vi "Day9-1.vi"() -> ()   [LabVIEW 2021]
panel:
  out "Tail pos":cluster{"x":i32, "y":i32}[](array[cluster])
  out "Head pos":cluster{"x":i32, "y":i32}[](array[cluster])
  out "size":i32
  out "Array":string[](array[string])
  out "array":string[][](array[string])
  in  "Tail":cluster{"x":i32, "y":i32}
  in  "Head":cluster{"x":i32, "y":i32}
  out "tail position":cluster{"x":i32, "y":i32}
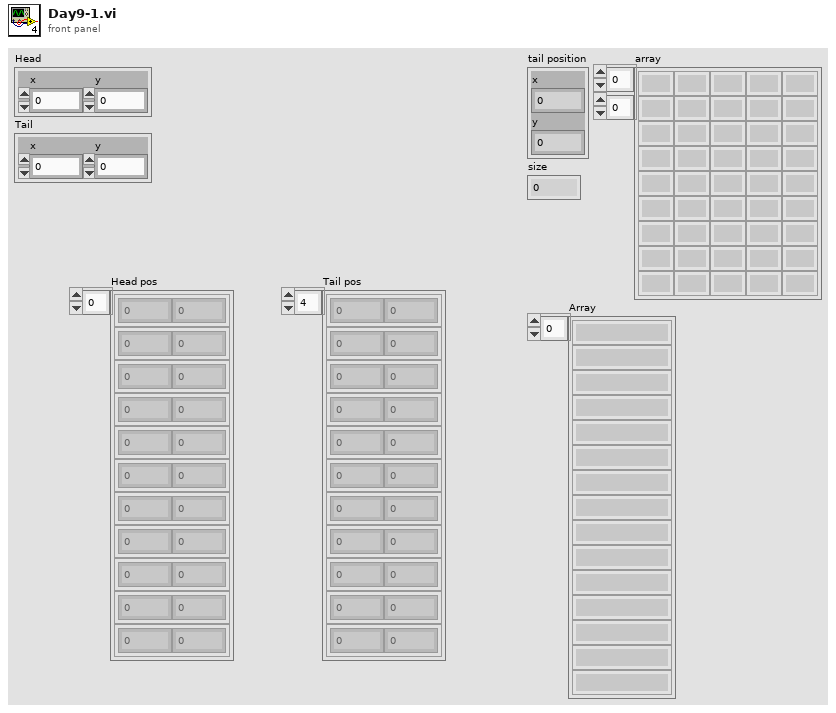
[diagram p1: front panel]
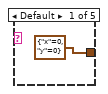
[diagram p2: hidden frame]
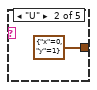
[diagram p3: hidden frame]
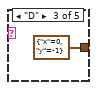
[diagram p4: hidden frame]
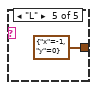
[diagram p5: hidden frame]
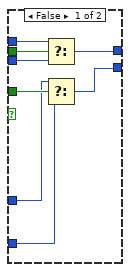
[diagram p6: hidden frame]
diagram:
  w8 = set{cluster{"x":i32, "y":i32}} {}  # Size: 0
  # "Initial starting position of Head and Tail = (0,0)"
  n1 = Spreadsheet String To Array(delimiter (Tab)=" ", format string="%s", spreadsheet string="R 2\nD 2\nR 2\nU 1\nR 2\nL 2\nD 1\nL 1\nD 2\nR 2\nU 2\nD 1\nR 2\nD 2\nU 1\nR 1\nD 1\nL 1\nU 1\nR 1\nL 1\nR 2\nU 2\nD 2\nR 2\nL 2\nU 1\nL 2\nU 2\nL 2\nR 2\nU 2\nR 1\nU 2\nL 2\nD 1\nR 1\nU 2\nD 2\nR 2\nL 2\nU 1\nD 1\nL 2\nU 2\nL 2\nU 1\nD 2\nR 1\nD 1\nR 2\nU 1\nL 2\nD 1\nU 2\nR 2\nL 1\nD 2\nU 1\nD 1\nL 1\nU 1\nR 1\nD 1\nR 1\nU 1\nD 2\nL 1\nD 1\nR 2\nD 1\nU 2\nD 2\nU 2\nL 1\nU 2\nR 2\nL 2\nD 2\nR 1\nL 2\nU 2\nL 1\nU 1\nL 1\nR 2\nL 2\nR 1\nD 1\nU 1\nL 2\nR 1\nL 1\nU 1\nD 1\nU 1\nD 1\nR 1\nL 2\nR 2\nL 1\nU 1\nD 2\nU 2\nL 2\nR 2\nU 1\nR 2\nL 2\nR 2\nL 1\nU 3\nD 1\nL 1\nD 3\nU 1\nD 2\nL 1\nR 3\nD 2\nU 3\nR 1\nD 3\nR 2\nD 1\nU 3\nL 1\nR 2\nL 3\nD 3\nU 2\nL 2\nR 3\nU 3\nD 3\nL 3\nD 2\nL 3\nR 1\nL 1\nD 1\nU 3\nD 3\nU 2\nL 3\nR 3\nU 1\nD 2\nR 2\nL 2\nD 3\nR 3\nU 1\nR 1\nL 3\nU 2\nL 2\nU 1\nR 1\nD 1\nR 3\nU 2\nD 1\nL 1\nU 1\nR 2\nL 1\nR 3\nL 1\nU 3\nL 2\nD 2\nL 2\nD 3\nL 2\nR 1\nU 2\nL 3\nD 1\nL 3\nD 1\nU 2\nL 3\nR 2\nU 1\nL 3\nD 3\nR 3\nU 2\nR 2\nD 3\nR 3\nU 2\nR 2\nL 2\nU 3\nR 1\nL 2\nD 3\nU 1\nL 1\nU 1\nL 2\nR 3\nL 3\nD 3\nR 3\nU 3\nL 1\nR 2\nD 3\nU 1\nR 2\nU 1\nD 1\nL 1\nD 2\nL 2\nD 3\nU 2\nD 1\nU 3\nD 3\nU 3\nR 3\nL 3\nU 4\nL 3\nD 1\nR 4\nU 3\nD 2\nR 1\nD 4\nL 3\nU 1\nL 1\nR 2\nD 1\nR 3\nD 3\nL 3\nD 4\nL 3\nR 4\nU 3\nR 3\nD 1\nR 3\nD 3\nR 3\nD 4\nU 4\nR 2\nD 3\nR 3\nD 2\nU 1\nR 2\nD 2\nU 2\nD 3\nL 2\nR 4\nD 4\nU 4\nR 3\nU 4\nR 1\nU 2\nR 4\nD 2\nL 4\nR 4\nU 3\nL 2\nU 2\nL 3\nR 3\nL 1\nU 4\nL 3\nU 3\nL 3\nU 1\nR 2\nU 3\nR 2\nL 3\nU 1\nD 3\nR 4\nD 1\nR 2\nL 1\nD 1\nU 2\nD 3\nR 4\nU 1\nL 3\nR 4\nU 4\nL 4\nR 2\nD 1\nU 4\nR 1\nD 3\nL 3\nD 1\nR 3\nD 2\nU 2\nL 1\nU 2\nD 3\nL 1\nU 3\nD 3\nL 3\nU 2\nL 3\nU 2\nR 1\nD 1\nR 1\nL 1\nD 2\nR 3\nD 2\nL 2\nR 3\nD 5\nR 5\nU 4\nD 5\nU 5\nD 4\nR 4\nD 2\nR 5\nL 4\nR 2\nL 2\nR 5\nU 5\nR 1\nD 2\nR 1\nL 3\nD 5\nU 3\nD 4\nR 3\nU 4\nD 1\nU 4\nL 5\nR 1\nU 4\nL 5\nU 3\nD 4\nL 2\nD 4\nU 4\nL 2\nD 1\nR 3\nD 1\nR 2\nD 4\nR 5\nL 1\nU 4\nL 4\nU 3\nL 1\nU 1\nR 4\nU 3\nL 1\nR 3\nD 5\nU 2\nR 4\nD 3\nL 2\nD 4\nR 5\nD 2\nU 3\nR 4\nD 4\nL 2\nU 4\nR 5\nL 1\nU 5\nD 1\nR 3\nL 4\nD 1\nU 3\nD 5\nR 2\nD 2\nL 5\nU 2\nD 3\nL 5\nD 5\nL 1\nR 5\nD 2\nU 3\nR 2\nL 2\nU 1\nL 5\nR 1\nL 4\nD 5\nR 5\nD 2\nU 5\nL 5\nD 1\nL 1\nD 3\nR 1\nD 2\nL 2\nR 4\nU 5\nL 2\nR 1\nU 3\nD 1\nU 1\nD 5\nR 2\nD 2\nR 3\nD 6\nU 1\nR 6\nD 4\nU 1\nR 5\nL 6\nR 2\nL 6\nU 6\nR 5\nD 2\nU 1\nD 2\nL 2\nD 5\nR 3\nU 4\nD 2\nL 1\nU 1\nD 3\nU 1\nD 1\nR 5\nU 1\nR 1\nD 3\nU 5\nL 6\nR 3\nL 6\nU 4\nD 2\nR 1\nL 6\nR 2\nD 3\nU 2\nR 2\nL 1\nD 1\nU 1\nR 4\nU 1\nR 2\nU 2\nL 2\nU 2\nD 5\nL 4\nU 6\nL 3\nD 6\nU 5\nL 6\nU 3\nR 5\nU 2\nR 4\nL 6\nD 1\nR 5\nD 4\nL 2\nR 2\nU 1\nD 2\nL 2\nU 4\nR 1\nD 2\nU 2\nR 6\nL 2\nD 5\nR 5\nL 3\nD 1\nU 1\nL 2\nD 4\nR 6\nL 5\nR 3\nU 1\nR 3\nL 1\nR 3\nU 1\nL 1\nU 4\nD 4\nU 3\nR 3\nU 1\nR 2\nD 1\nL 6\nU 2\nR 2\nD 1\nR 5\nL 2\nD 5\nL 3\nR 6\nD 2\nL 2\nD 3\nL 5\nD 7\nL 7\nD 4\nU 5\nR 7\nL 7\nD 3\nU 5\nR 6\nU 3\nL 6\nR 5\nL 4\nD 4\nR 4\nL 6\nD 6\nU 3\nD 3\nR 7\nU 1\nL 5\nU 3\nL 4\nU 3\nL 5\nD 1\nR 7\nU 3\nL 6\nD 1\nU 3\nL 2\nU 6\nL 6\nD 1\nU 1\nD 2\nL 5\nU 4\nR 5\nD 7\nU 3\nD 4\nL 1\nD 3\nR 7\nD 2\nU 4\nL 1\nD 3\nR 3\nD 6\nR 4\nU 3\nD 4\nR 6\nL 7\nU 5\nL 7\nR 3\nL 7\nD 5\nR 7\nD 4\nU 3\nR 6\nU 7\nD 2\nR 2\nL 2\nD 1\nR 3\nU 3\nD 5\nU 3\nL 3\nD 6\nL 6\nR 1\nL 5\nD 6\nU 4\nR 2\nL 2\nD 1\nU 7\nL 5\nD 3\nU 1\nL 1\nR 1\nL 6\nR 1\nD 6\nU 4\nL 7\nU 6\nR 6\nL 2\nD 5\nR 1\nD 6\nL 1\nR 3\nD 1\nU 5\nL 1\nD 3\nU 7\nD 5\nU 7\nD 7\nU 4\nR 3\nU 4\nL 8\nU 1\nR 1\nD 2\nU 5\nD 2\nL 5\nD 6\nU 4\nR 5\nL 5\nU 7\nL 3\nD 1\nL 2\nR 8\nL 1\nU 8\nL 2\nD 3\nR 6\nL 8\nD 2\nL 1\nU 4\nD 1\nR 2\nD 7\nU 5\nD 4\nU 4\nL 2\nD 6\nU 1\nD 5\nU 2\nD 2\nL 8\nD 6\nL 2\nU 1\nR 7\nD 1\nU 5\nL 6\nD 3\nL 2\nD 8\nR 6\nL 5\nU 2\nL 6\nU 4\nD 6\nL 7\nU 8\nL 5\nD 8\nR 8\nD 6\nL 3\nU 6\nL 1\nD 8\nR 7\nL 7\nR 2\nD 6\nR 1\nU 5\nL 5\nR 5\nL 3\nU 8\nL 1\nU 2\nD 5\nR 8\nU 5\nL 5\nD 2\nR 5\nU 1\nD 8\nR 3\nU 1\nR 6\nD 6\nR 5\nD 6\nL 8\nU 8\nL 8\nU 8\nL 8\nR 8\nU 8\nR 5\nL 1\nD 3\nU 1\nD 6\nU 1\nL 8\nU 3\nR 5\nL 2\nR 1\nD 2\nL 2\nU 4\nD 1\nR 1\nD 2\nR 2\nU 4\nR 3\nU 8\nD 9\nL 9\nD 5\nL 4\nD 7\nL 9\nU 4\nL 9\nD 7\nU 4\nL 3\nU 2\nR 5\nU 3\nL 1\nR 5\nL 8\nU 4\nR 6\nL 8\nU 1\nR 7\nD 6\nR 6\nU 7\nL 9\nR 7\nU 8\nR 5\nU 6\nL 4\nD 4\nL 3\nR 8\nU 6\nL 7\nR 4\nD 7\nR 3\nL 3\nD 2\nL 2\nU 5\nR 8\nL 7\nR 9\nD 8\nU 1\nL 1\nD 4\nU 6\nR 4\nL 2\nR 9\nL 9\nR 2\nD 3\nL 4\nU 6\nR 3\nD 5\nL 4\nR 8\nU 3\nR 5\nL 3\nD 7\nR 1\nD 2\nU 5\nL 7\nD 6\nR 1\nD 9\nL 9\nR 8\nU 8\nL 8\nD 7\nU 3\nL 2\nU 4\nD 8\nU 6\nR 3\nU 5\nR 7\nD 1\nR 8\nL 9\nU 7\nD 9\nL 2\nR 7\nU 1\nR 6\nD 3\nL 5\nU 10\nL 8\nR 3\nL 4\nD 9\nU 4\nL 5\nU 5\nD 10\nR 8\nU 6\nL 3\nU 4\nD 6\nL 8\nD 2\nR 8\nL 9\nU 3\nR 5\nD 1\nR 9\nD 6\nL 5\nR 10\nL 8\nR 9\nL 6\nU 8\nL 8\nU 5\nR 3\nU 6\nD 3\nL 10\nD 9\nU 5\nL 3\nU 6\nR 2\nD 7\nR 9\nL 5\nD 3\nU 3\nR 2\nD 10\nU 3\nR 2\nU 6\nL 10\nR 3\nU 3\nR 4\nL 8\nR 1\nL 6\nU 9\nL 7\nD 7\nR 6\nU 3\nR 1\nL 6\nD 5\nL 3\nU 2\nL 5\nR 9\nD 5\nR 4\nL 2\nU 5\nD 7\nL 10\nD 9\nU 7\nD 9\nR 5\nD 3\nL 1\nR 10\nL 4\nU 6\nR 7\nL 2\nR 6\nL 3\nR 3\nD 2\nL 1\nR 2\nL 7\nD 8\nR 5\nL 7\nD 8\nU 5\nL 8\nU 4\nR 8\nU 1\nD 1\nU 4\nD 6\nR 8\nU 10\nD 5\nU 5\nL 1\nD 2\nR 10\nU 10\nR 2\nL 9\nR 2\nD 3\nL 6\nR 10\nD 10\nR 9\nD 7\nU 3\nR 4\nD 9\nR 4\nD 9\nU 9\nL 8\nD 7\nR 7\nU 7\nR 7\nD 9\nL 7\nU 5\nL 10\nR 8\nL 11\nD 9\nL 5\nR 11\nL 6\nR 1\nU 2\nD 9\nL 3\nR 6\nL 6\nR 2\nL 6\nD 6\nR 2\nD 5\nL 8\nR 9\nU 6\nD 6\nL 1\nR 3\nD 2\nR 5\nD 6\nL 1\nD 10\nU 2\nR 4\nU 6\nR 11\nD 1\nR 2\nL 4\nD 9\nL 4\nU 8\nD 10\nU 4\nR 10\nD 1\nU 11\nR 2\nL 11\nD 7\nU 1\nL 7\nU 10\nD 10\nL 11\nR 1\nU 8\nR 1\nL 11\nR 3\nD 10\nR 10\nL 9\nU 7\nR 9\nL 6\nR 7\nU 5\nR 6\nU 4\nL 11\nU 7\nR 7\nL 4\nU 4\nR 2\nD 3\nR 2\nL 9\nD 4\nL 11\nR 6\nD 2\nL 9\nR 7\nD 6\nU 5\nL 8\nD 9\nR 11\nU 11\nR 6\nD 11\nL 9\nR 4\nL 6\nU 10\nR 11\nU 5\nL 6\nR 12\nD 3\nR 4\nU 12\nR 6\nD 8\nR 1\nD 2\nL 11\nR 6\nD 5\nU 10\nD 5\nR 8\nL 6\nD 5\nU 5\nR 8\nL 1\nD 10\nR 5\nU 6\nL 8\nR 4\nL 10\nD 6\nR 3\nD 9\nL 4\nR 9\nU 5\nR 2\nU 11\nR 9\nU 8\nR 7\nL 2\nD 7\nU 7\nD 8\nU 12\nR 6\nD 12\nR 5\nD 10\nU 2\nD 8\nU 6\nR 3\nU 5\nR 5\nL 11\nD 10\nR 3\nU 11\nD 8\nR 7\nL 3\nU 9\nR 4\nL 2\nD 4\nR 8\nD 9\nR 2\nD 3\nU 6\nL 5\nD 4\nL 2\nR 9\nU 5\nD 1\nU 9\nR 9\nU 11\nL 12\nR 10\nD 5\nU 1\nR 9\nU 4\nD 8\nR 1\nD 5\nR 7\nU 11\nL 6\nU 1\nR 12\nD 1\nR 7\nU 12\nD 9\nR 12\nL 1\nU 3\nD 6\nR 11\nL 6\nU 8\nD 11\nR 7\nU 5\nD 4\nU 1\nL 11\nD 1\nU 5\nR 13\nL 9\nU 4\nD 4\nR 10\nU 4\nD 7\nL 4\nD 10\nR 6\nD 5\nR 9\nL 10\nD 2\nU 11\nD 8\nU 1\nR 8\nU 5\nR 8\nD 10\nL 10\nD 7\nR 5\nU 6\nD 7\nU 9\nR 8\nD 4\nR 2\nD 1\nL 1\nU 2\nR 10\nD 2\nU 13\nL 9\nU 13\nL 12\nU 12\nD 6\nL 1\nR 4\nL 7\nR 4\nL 2\nU 8\nR 7\nD 10\nU 2\nL 8\nD 5\nR 9\nD 9\nR 2\nL 3\nU 2\nD 11\nU 5\nD 12\nR 3\nU 10\nD 2\nR 1\nD 13\nU 7\nL 7\nR 1\nU 1\nR 1\nU 6\nD 12\nR 7\nL 7\nR 9\nU 10\nR 13\nD 3\nR 12\nU 1\nL 6\nR 9\nU 10\nL 1\nU 13\nR 2\nD 8\nU 12\nD 10\nL 7\nU 6\nD 9\nL 11\nD 8\nU 4\nR 1\nD 11\nL 8\nU 1\nD 4\nR 7\nU 7\nR 5\nL 1\nR 14\nL 8\nD 10\nR 13\nU 13\nR 9\nL 13\nU 2\nD 7\nR 11\nD 2\nL 9\nD 11\nL 2\nU 12\nD 11\nR 12\nD 3\nR 6\nL 11\nR 7\nD 3\nU 6\nD 9\nL 10\nR 13\nD 7\nU 14\nL 10\nR 11\nD 12\nR 12\nU 13\nR 4\nL 14\nU 5\nL 4\nU 10\nL 3\nU 13\nR 9\nD 7\nU 8\nR 5\nL 14\nU 5\nR 6\nD 13\nL 13\nU 9\nR 13\nD 1\nL 8\nR 9\nU 8\nL 7\nU 4\nD 4\nR 4\nL 5\nU 11\nR 14\nL 2\nU 1\nD 14\nR 13\nD 3\nL 13\nD 2\nU 9\nD 14\nU 1\nR 1\nD 12\nL 6\nR 4\nU 4\nL 11\nU 14\nD 13\nR 12\nL 7\nU 13\nR 4\nU 14\nL 14\nR 11\nL 8\nD 3\nU 4\nR 1\nU 5\nD 12\nL 5\nU 14\nD 6\nR 6\nU 4\nL 1\nD 11\nU 9\nR 5\nU 13\nD 7\nL 5\nD 3\nL 8\nU 7\nD 4\nL 13\nR 1\nD 11\nL 7\nU 6\nD 9\nR 10\nD 6\nR 9\nL 2\nD 6\nU 12\nL 10\nD 3\nU 6\nL 4\nR 4\nU 12\nD 13\nR 9\nL 1\nR 5\nU 14\nR 14\nD 7\nU 10\nR 3\nL 4\nU 6\nL 13\nU 14\nR 10\nL 7\nD 12\nU 5\nL 11\nD 7\nU 9\nD 4\nL 1\nR 11\nD 9\nL 5\nD 15\nR 4\nU 12\nL 1\nU 8\nL 15\nD 15\nL 3\nR 11\nL 9\nR 1\nU 12\nD 9\nR 7\nD 6\nU 2\nL 12\nU 13\nR 11\nL 15\nD 4\nL 8\nU 6\nL 7\nR 2\nU 7\nD 2\nU 13\nD 10\nL 13\nU 1\nD 6\nL 11\nR 14\nL 5\nU 2\nR 11\nD 10\nL 4\nR 14\nU 13\nD 9\nU 2\nD 4\nR 14\nL 4\nR 4\nL 4\nU 6\nD 11\nL 10\nU 9\nL 3\nU 12\nL 8\nU 9\nD 4\nU 4\nL 10\nU 1\nD 8\nU 15\nD 3\nU 12\nR 3\nD 8\nU 1\nR 10\nL 1\nU 5\nD 1\nL 1\nR 3\nU 1\nR 8\nU 10\nR 1\nU 11\nR 15\nD 16\nU 13\nD 7\nU 7\nD 14\nR 9\nL 13\nR 12\nU 2\nR 11\nL 11\nR 3\nD 11\nU 11\nR 2\nD 3\nU 6\nL 14\nR 6\nL 6\nU 3\nR 3\nD 1\nU 5\nL 3\nR 4\nD 9\nU 15\nR 2\nU 5\nD 5\nR 14\nU 6\nR 1\nD 4\nU 2\nD 3\nR 8\nL 4\nD 2\nU 12\nD 2\nU 7\nL 14\nU 1\nR 10\nL 4\nD 12\nL 9\nD 16\nU 2\nR 7\nD 16\nU 9\nD 13\nU 7\nL 14\nD 5\nR 12\nU 13\nR 13\nU 2\nL 11\nD 9\nU 2\nR 8\nU 5\nR 7\nU 9\nL 11\nD 16\nU 10\nR 5\nD 7\nL 6\nD 8\nU 4\nR 3\nD 5\nL 5\nU 11\nR 4\nD 12\nR 12\nL 10\nR 15\nU 9\nD 12\nL 11\nU 6\nD 11\nU 12\nL 6\nR 3\nU 12\nD 5\nL 1\nR 12\nU 14\nL 1\nD 2\nL 4\nD 7\nL 12\nU 10\nL 12\nU 4\nD 14\nR 13\nU 9\nL 2\nU 6\nL 1\nU 9\nD 16\nL 2\nR 16\nD 5\nL 7\nU 13\nL 15\nR 1\nD 8\nR 15\nD 5\nR 12\nL 5\nR 11\nU 17\nD 13\nU 13\nL 4\nD 8\nL 1\nD 7\nR 11\nU 7\nR 11\nL 9\nD 3\nL 2\nU 4\nD 16\nL 10\nU 11\nR 5\nU 4\nR 6\nL 11\nR 17\nU 13\nR 12\nD 11\nL 17\nU 15\nD 4\nR 9\nU 9\nL 10\nD 5\nR 14\nU 10\nR 5\nU 15\nL 12\nD 14\nR 14\nL 11\nR 5\nU 7\nD 1\nR 4\nD 14\nU 3\nR 6\nD 5\nR 1\nD 12\nL 14\nD 6\nL 15\nU 16\nD 10\nR 12\nD 9\nU 1\nD 1\nL 4\nD 6\nU 16\nR 11\nL 11\nR 3\nL 2\nU 12\nR 9\nD 16\nR 12\nL 14\nU 6\nL 7\nD 5\nU 4\nR 13\nL 8\nD 16\nU 5\nD 5\nU 6\nR 14\nL 6\nD 7\nU 3\nL 15\nR 14\nL 17\nR 17\nU 16\nL 4\nR 3\nU 1\nD 15\nL 12\nD 11\nL 18\nD 18\nU 10\nD 4\nU 1\nR 11\nU 18\nD 12\nR 11\nU 13\nD 14\nR 17\nD 18\nU 13\nR 8\nU 4\nR 9\nD 18\nL 6\nR 7\nL 14\nU 10\nL 10\nU 16\nD 15\nL 15\nD 3\nL 2\nD 7\nR 3\nD 7\nU 11\nL 6\nR 8\nL 3\nU 3\nR 8\nD 8\nU 10\nL 15\nD 1\nU 16\nR 1\nL 13\nR 7\nU 10\nL 12\nR 8\nD 3\nL 14\nD 12\nR 12\nD 3\nL 2\nD 15\nR 3\nL 14\nD 4\nR 5\nL 13\nD 9\nU 2\nL 5\nR 13\nD 4\nL 14\nR 14\nD 16\nR 1\nU 11\nR 6\nL 7\nU 16\nL 15\nD 6\nU 7\nR 16\nD 2\nL 15\nD 18\nU 3\nD 1\nR 7\nD 1\nL 4\nD 16\nU 12\nL 12\nR 7\nU 5\nL 5\nU 13\nR 13\nU 7\nL 9\nR 9\nU 8\nD 6\nL 3\nU 4\nR 12\nL 12\nD 16\nU 12\nL 4\nR 11\nU 9\nD 13\nR 15\nL 3\nD 17\nR 6\nD 13\nR 6\nD 5\nL 19\nU 10\nD 3\nL 2\nU 13\nR 2\nD 3\nL 3\nU 3\nR 1\nU 12\nL 2\nD 19\nL 17\nR 10\nD 11\nU 8\nR 10\nL 15\nR 4\nD 9\nU 4\nD 11\nU 4\nD 3\nL 5\nD 15\nU 1\nL 19\nD 16\nR 11\nU 12\nD 16\nL 4\nR 13\nU 2\nL 19\nU 9\nR 5\nD 7\nR 19\nL 9\nU 2\nD 2\nR 3\nU 10\nL 13\nD 16\nL 2\nD 5\nL 8\nR 9\nL 18\nR 9\nU 13\nD 7\nR 14\nU 8\nR 18\nL 18\nU 8\nL 13\nR 9\nU 5\nL 16\nU 4\nD 4\nR 10\nU 13\nR 2\nL 6\nR 18\nD 3\nL 11\nR 12\nL 2\nR 12\nD 7\nU 12\nR 13\nU 14\nD 1\nR 8\nL 13\nU 5\nL 9\nU 19\nD 14\nL 4\nU 8\nD 8\nU 1\nD 16\nU 4\nD 8\nU 20", array type (2D Dbl)=string[][] []) -> (array=w11:string[][])
  "array" <- w11
  n2 = for {
    tunnel: w11 -> [w21] mode=indexing
    tunnel: [w17] -> w5 mode=concatenating
    n3 = Index Array(array=w21) -> (element #1=w18:string, element #2=w20:string)  [unwired: 2 in]
    n4 = Decimal String To Number(string=w20) -> (number=w19:i32)  [unwired: 2 in, 1 out]
    n5 = Initialize Array(w18, w19) -> (w17:string[])
  }
  "Array" <- w5
  n6 = for {
    shift-right: [w26] -> w16
    shift-left: "Tail" -> [w36]
    tunnel: [w26] -> w10 mode=indexing
    tunnel: w5 -> [w25] mode=indexing
    shift-right: [w22] -> _
    shift-left: "Head" -> [w23]
    tunnel: [w22] -> w4 mode=indexing
    w47 = 2 ("y")
    n7 = case shown="\"R\"" w25 {
      tunnel: [cluster{"x":i32, "y":i32} {"x"=0, "y"=0} ("Tail") cluster{"x":i32, "y":i32} {"x"=0, "y"=1} ("Tail") cluster{"x":i32, "y":i32} {"x"=0, "y"=-1} ("Tail") cluster{"x":i32, "y":i32} {"x"=1, "y"=0} ("Tail") cluster{"x":i32, "y":i32} {"x"=-1, "y"=0} ("Tail")] -> w24
      frame Default {
      }
      frame "U" {
      }
      frame "D" {
      }
      frame "R" {
      }
      frame "L" {
      }
    }
    n8 = Add(x=w24, y=w23) -> (x+y=w22:cluster{"x":i32, "y":i32})
    n9 = Subtract(x=w22, y=w36) -> (x-y=w33:cluster{"x":i32, "y":i32})
    n10 = Square(x=w33) -> (x^2=w32:cluster{"x":i32, "y":i32})
    n11 = Unbundle By Name(w33) -> ("x"=w46:i32, "y"=w44:i32)
    n12 = Unbundle By Name(w36) -> ("x"=w40:i32, "y"=w37:i32)
    n13 = Absolute Value(x=w46) -> (abs(x)=w49:i32)
    n14 = Absolute Value(x=w44) -> (abs(x)=w48:i32)
    n15 = Unbundle(w32) -> ("x"=w31:i32, "y"=w30:i32)
    n16 = Greater Or Equal?(x=w49, y=w47) -> (x >= y?=w42:bool)
    n17 = Greater Or Equal?(x=w48, y=w47) -> (x >= y?=w39:bool)
    n18 = Add(x=w31, y=w30) -> (x+y=w29:i32)
    n19 = Sign(1:w46) -> (0:w45:i32)
    n20 = Sign(1:w44) -> (0:w43:i32)
    n21 = Greater Or Equal?(x=w29, y=5) -> (x >= y?=w27:bool)
    n22 = Add(x=w45, y=w40) -> (x+y=w41:i32)
    n23 = Add(x=w43, y=w37) -> (x+y=w38:i32)
    n24 = case shown="True" w27 {
      tunnel: w42 -> [w62 _]
      tunnel: w41 -> [w61 w64]
      tunnel: w40 -> [w60 _]
      tunnel: w39 -> [w59 _]
      tunnel: w38 -> [w58 w63]
      tunnel: w37 -> [w57 _]
      tunnel: [w56 w64] -> w35
      tunnel: [w55 w63] -> w34
      frame False {
        n25 = Select(t=w61, s=w62, f=w60) -> (s? t:f=w56:i32)
        n26 = Select(t=w58, s=w59, f=w57) -> (s? t:f=w55:i32)
      }
      frame True {
      }
    }
    n27 = Bundle By Name(cluster=w36, "x"=w35, "y"=w34) -> (w26:cluster{"x":i32, "y":i32})
  }
  "tail position" <- w16
  n28 = Build Array (concatenate)("Head", w4) -> (→"Head pos":cluster{"x":i32, "y":i32}[])
  n29 = Build Array (concatenate)("Tail", w10) -> (w1:cluster{"x":i32, "y":i32}[])
  "Tail pos" <- w1
  n30 = for {
    tunnel: w1 -> [w66] mode=indexing
    shift-right: [w65] -> w7
    shift-left: w8 -> [w67]
    n31 = Insert Into Set(10:w66, 11:w67) -> (3:w65:set{cluster{"x":i32, "y":i32}})  [unwired: 1 out]
  }
  n32 = Collection Size(1:w7) -> (0:→"size":i32)
